vi "Do.vi"(8 "error in (no error)":errorcluster, 10 "Actor in":refnum<class "Actor.lvclass">, 11 "Display All Users In Manager Msg":refnum<class "Display All Users In Manager Msg.lvclass">) -> (0 "error out":errorcluster, 2 "Actor out":refnum<class "Actor.lvclass">)   [LabVIEW 2017, in "User Manager View.lvlib" / "Display All Users In Manager Msg.lvclass"]
doc: "This VI delivers the message to the actor by calling the appropriate method(s) on the actor."
uses:
  <vilib>/gpm_packages/@cs/User Manager App/User Manager View/User Manager View Messages/Display All Users In Manager Msg/Display All Users In Manager Msg.lvclass
  <vilib>/ActorFramework/Actor/Actor.lvclass
  <vilib>/gpm_packages/@cs/User Manager App/User Manager View/User Manager View/User Manager View.lvclass
  C:/Program Files/National Instruments/LabVIEW 2017/vi.lib/ActorFramework/Actor/Actor.lvclass
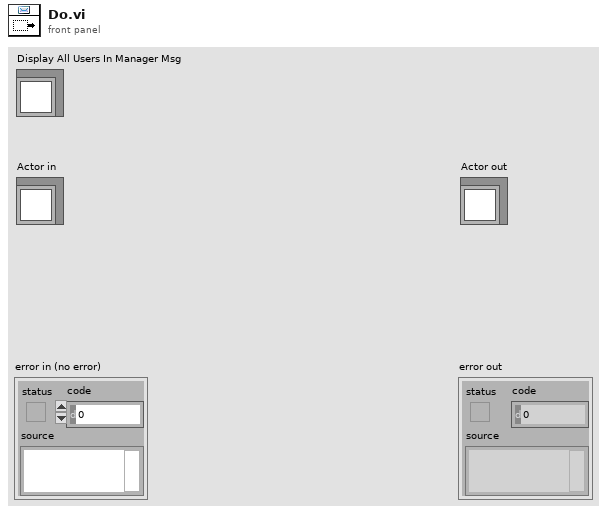
[diagram p1: front panel]
types:
  T1 = typedef "User Manager Application Types.lvlib/New User Information.ctl" = cluster{"User Info":T2, "User Level":T3}
  T2 = typedef "User Manager Application Types.lvlib/Credentials.ctl" = cluster{"Username":string, "Password":string}
  T3 = typedef "User Manager Application Types.lvlib/User Levels.ctl" = cluster{"Rank":i32, "Title":string}
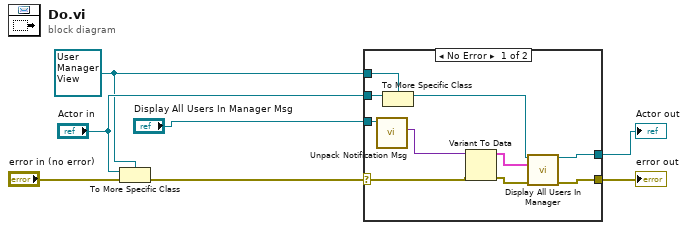
[diagram p0: block diagram]
diagram:
  w2 = refnum<class "User Manager View.lvclass"> refnum ("Actor in")
  n1 = To More Specific Class(target class=w2, reference="Actor in", error in="error in (no error)") -> (error out=w6:errorcluster)  [unwired: 1 out]
  n2 = case shown="No Error" w6 {
    selector: w6 -> [w11 w19]
    tunnel: [w17 w19] -> w5
    tunnel: [w16 w18] -> w4
    tunnel: "Actor in" -> [w15 w18]
    tunnel: w2 -> [w14 _]
    tunnel: "Display All Users In Manager Msg" -> [w12 _]
    frame No Error {
      n3 = call-dynamic "Unpack Notification Msg.vi"("Notification Msg"=w12) -> ("Value"=w9:variant)  [unwired: 8 in, 2 out]
      n4 = To More Specific Class(target class=w14, reference=w15) -> (specific class reference=w13:refnum<class "User Manager View.lvclass">)  [unwired: 1 in, 1 out]
      n5 = Variant To Data(error in=w11, Variant=w9) -> (data=w8:T1[], error out=w10:errorcluster)  [unwired: 1 in]
      n6 = call-dynamic "Display All Users In Manager.vi"("User Manager View in"=w13, "All Users In Manager"=w8, "error in (no error)"=w10) -> ("User Manager View out"=w16:refnum<class "User Manager View.lvclass">, "error out"=w17:errorcluster)  [unwired: 11 in]
    }
    frame Error {
      # "If type check fails, pass the original object out again."
    }
  }
  "error out" <- w5
  "Actor out" <- w4
